vi "Set Hardware Relay State.vi"(0 "DevicePropertyRelay in":refnum<class "DevicePropertyRelay.lvclass">, 5 "session in":refnum<k21>, 7 "device in":refnum<k21>, 9 "relay action (Close Relay)":T1=21 caption="relay action" items=["CloseRelay"=21, "OpenRelay"=20], 11 "error in (no error)":errorcluster) -> (4 "DevicePropertyRelay out":refnum<class "DevicePropertyRelay.lvclass">, 6 "session out":refnum<k21>, 8 "device out":refnum<k21>, 15 "error out":errorcluster)   [LabVIEW 2015, in "DevicePropertyRelay.lvclass"]
doc: "This uses a device property and/or command to set the current hardware state of a relay."
uses:
  DevicePropertyRelay.lvclass
  slscsl/RelayAction.ctl
  DevicePropertyRelay.lvclass/DevicePropertyRelay.ctl
  <vilib>/SLSC/Set Device Property (Bool).vi
  <vilib>/SLSC/Commit Properties for Devices.vi
  <vilib>/SLSC/Execute Device Command.vi
  Relay Interface/RelayInterface.lvclass
  <vilib>/SLSC/SLSC.lvlib
  slscsl/slscsl.lvclass
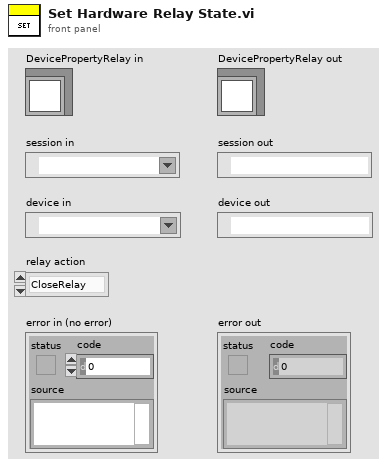
[diagram p1: front panel]
types:
  T1 = typedef "slscsl.lvclass/RelayAction.ctl" = u16
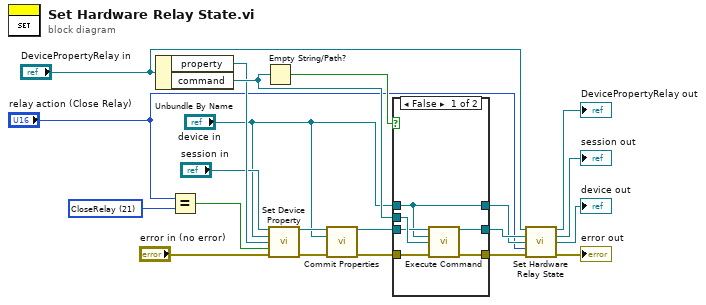
[diagram p0: block diagram]
diagram:
  w1 = T1 21 items=["CloseRelay"=21, "OpenRelay"=20] ("RelayAction")
  n1 = Unbundle By Name("DevicePropertyRelay in") -> ("property"=w16:refnum<k21>, "command"=w21:refnum<k21>)
  n2 = Equal?(x="relay action (Close Relay)", y=w1) -> (x = y?=w19:bool)
  n3 = Empty String/Path?(string/path=w21) -> (empty?=w20:bool)
  n4 = call-poly <vilib>:"Set Device Property.vi"("session in"="session in", "devices"="device in", "property"=w16, "property value"=w19, "error in (no error)"="error in (no error)") -> ("session out"=w18:refnum<k21>, "error out"=w17:errorcluster)  [unwired: 9 in]
  n5 = call-poly <vilib>:"Commit Properties.vi"("session in"=w18, "devices"="device in", "error in (no error)"=w17) -> ("session out"=w15:refnum<k21>, "error out"=w13:errorcluster)  [unwired: 11 in]
  n6 = case shown="False" w20 {
    tunnel: w21 -> [w27 _]
    tunnel: "device in" -> [w22 w28]
    tunnel: w15 -> [w26 w30]
    tunnel: [w25 w30] -> w4
    tunnel: w13 -> [w24 w29]
    tunnel: [w23 w29] -> w8
    tunnel: [w22 w28] -> w3
    frame False {
      n7 = call-poly <vilib>:"Execute Command.vi"("session in"=w26, "devices"=w22, "command"=w27, "error in (no error)"=w24) -> ("session out"=w25:refnum<k21>, "error out"=w23:errorcluster)  [unwired: 10 in]
    }
    frame True {
    }
  }
  n8 = call-parent "Set Hardware Relay State.vi"("RelayInterface in"="DevicePropertyRelay in", "session in"=w4, "device in"=w3, "relay action (Close Relay)"="relay action (Close Relay)", "error in (no error)"=w8) -> ("RelayInterface out"=→"DevicePropertyRelay out":refnum<class "DevicePropertyRelay.lvclass">, "session out"=→"session out":refnum<k21>, "device out"=→"device out":refnum<k21>, "error out"=→"error out":errorcluster)  [unwired: 7 in]
